vi "Create Evaluation String.vi"(8 "error in (no error)":errorcluster, 10 "Evaluation String":string, 11 "FP LT in":refnum<class "FP LT.lvclass">) -> (0 "error out":errorcluster, 3 "FP LT out":refnum<class "FP LT.lvclass">)   [LabVIEW 2018, in "FP LT.lvclass"]
uses:
  FP LT.lvclass
  C:/Users/UKHornP/Documents/Work/Projects/Assert_API/Plugins/Utility/Test Classes/Test.lvclass
  Floating Point.lvclass
  Test.lvclass
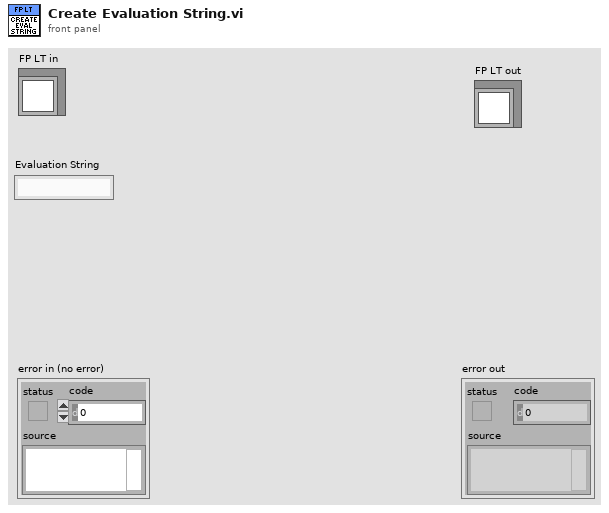
[diagram p1: front panel]
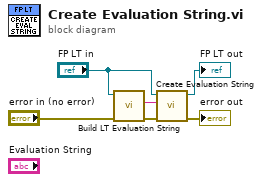
[diagram p0: block diagram]
diagram:
  n1 = call "Build LT Evaluation String.vi"("error in (no error)"="error in (no error)", "Test in"="FP LT in") -> ("error out"=w3:errorcluster, "Equals Evaluation String"=w1:string)  [unwired: 8 in]
  n2 = call-parent "Create Evaluation String.vi"("error in (no error)"=w3, "Evaluation String"=w1, "Floating Point in"="FP LT in") -> ("error out"=→"error out":errorcluster, "Floating Point out"=→"FP LT out":refnum<class "FP LT.lvclass">)  [unwired: 7 in]
